vi "linearize_project.vi"() -> ()   [LabVIEW 2015]
uses:
  <vilib>/addons/Control Design/_Model Construction/Model Typedefs.llb/CD State Space Model (MIMO).ctl
  <vilib>/addons/Control Design/_Model Construction/Model Typedefs.llb/CD General Elements.ctl
  <vilib>/Simulation/Scripting/Companion Diagram/SimConfigNode/SimParams.ctl
  <vilib>/Simulation/Scripting/Companion Diagram/SimConfigNode/_simSolvers.ctl
  <vilib>/Simulation/Implementation/Shared/SIMSCR Execution Mode.ctl
  <vilib>/Simulation/Param Hierarchy/Typedefs/SIMPH Param Control Actions.ctl
  <vilib>/Simulation/Implementation/Shared/NILVSim_ParamChanged.vi
  <vilib>/Simulation/Implementation/Shared/NILVSIM_BeginStep.vi
  <vilib>/Simulation/DataSources/Implementation/NILVSim Step.llb/SIM Step (scalar).vi
  <vilib>/Simulation/ContinuousLinear/Implementation/NILVSim Transfer Function.llb/SIM Transfer Function Distributor (SISO CD).vi
  <vilib>/Simulation/ContinuousLinear/Implementation/NILVSim Transfer Function.llb/SIM Transfer Function Collector (SISO).vi
  <vilib>/Simulation/SignalDisplay/Implementation/NILVSim Time Waveform.llb/SIM Time Waveform (scalar).vi
  <vilib>/Simulation/Nonlinear/Implementation/NILVSim Saturation.llb/SIM Saturation (scalar).vi
  <vilib>/Simulation/Implementation/Shared/NILVSim_Manager.vi
  <vilib>/Utility/error.llb/Clear Errors.vi
  <vilib>/Simulation/Implementation/Shared/NILVSim_FinalizeModel.vi
  <vilib>/Simulation/Model Trim and Linearize/SIM Query Subsystem.llb/SIM Query Subsystem (Path).vi
  <vilib>/Simulation/Model Trim and Linearize/SIM Linearize.llb/SIM Linearize (Path).vi
  <vilib>/addons/Control Design/_Model Construction/Model Information.llb/Model Information SubVIs/cd_Get Matrices From SS Model.vi
  <vilib>/addons/Control Design/_Model Construction/Model Creation.llb/Model Creation SubVI/cd_Create State Space Model.vi
  <vilib>/addons/Control Design/_Model Conversions/Model Type.llb/Model Conversion SubVI/cd_Convert State-Space to Transfer Function Model.vi
  <vilib>/addons/Control Design/_Utility/Model Viewer.llb/Model Viewer SubVI/cd_Draw Transfer Function Equation (TF).vi
  <vilib>/addons/Control Design/_Model Construction/Model Creation.llb/Model Creation SubVI/cd_Create Transfer Function Model.vi
  <vilib>/addons/Control Design/_Model Interconnection/Model Interconnection.llb/Model Interconnection SubVI/cd_Add Models (TF and TF).vi
  <vilib>/Simulation/Implementation/Shared/SIM Unbundle Sim Info.vi
  <vilib>/Simulation/Implementation/Shared/NILVSim_Initialize.vi
  <vilib>/Simulation/Utility/Implementation/NILVSim Get Time and IsAcceptedStep.vi
  <vilib>/addons/control/pid/pid.llb/PID.vi
  <vilib>/addons/control/pid/pid.llb/PID (DBL).vi
  <vilib>/Simulation/Implementation/Shared/SIMSH Read Queue.vi
  <vilib>/Simulation/Implementation/Shared/NILVSim_GetModelError.vi
  <vilib>/Simulation/Implementation/Shared/SIM Bundle Sim Info.vi
  <vilib>/Simulation/Scripting/Companion Diagram/SimConfigNode/SimDog.xnode
  <vilib>/Simulation/Implementation/XNodeFramework/SimXNode/SimX.xnode
  <vilib>/addons/Control Design/_Model Construction/NI_LinSys_Model Information.lvlib
  <vilib>/addons/Control Design/_Model Construction/NI_LinSys_Model Creation.lvlib
  <vilib>/addons/Control Design/_Model Conversions/NI_CD_Model Type.lvlib
  <vilib>/addons/Control Design/_Utility/NI_CD_Model Viewer.lvlib
  <vilib>/addons/Control Design/_Model Interconnection/NI_CD_Model Interconnection.lvlib
  <vilib>/addons/Control Design/_Model Construction/NI_LinSys_Model Typedefs.lvlib
  <vilib>/addons/Control Design/_Model Construction/Model Typedefs.llb/CD Transfer Function Model (SISO).ctl
  <vilib>/addons/Control Design/_Model Construction/Model Typedefs.llb/CD Transfer Function Model (MIMO).ctl
  <vilib>/Simulation/ContinuousLinear/Implementation/NILVSim Transfer Function.llb/SIM Transfer Function (SISO CD).vi
  <vilib>/addons/control/pid/NI_PID_pid.lvlib
  <vilib>/Simulation/Implementation/Shared/NI_SIM_Implementation.lvlib
panel:
  in  "PID gains 2":T1={"proportional gain (Kc)"=1.0, "integral time (Ti, min)"=0.01, "derivative time (Td, min)"=0.0} {"derivative time (Td, min)" format="%.3f"; "integral time (Ti, min)" format="%.3f"; "proportional gain (Kc)" format="%.3f"}
  in  "set point 2":dbl
  in  "PID gains":T1={"proportional gain (Kc)"=1.0, "integral time (Ti, min)"=0.01, "derivative time (Td, min)"=0.0} {"derivative time (Td, min)" format="%.3f"; "integral time (Ti, min)" format="%.3f"; "proportional gain (Kc)" format="%.3f"}
  in  "set point1":dbl
  out "h2 2":waveform(dbl)(graph)
  out "h1 2":waveform(dbl)(graph)
  out "h2":waveform(dbl)(graph)
  out "h1":waveform(dbl)(graph)
  out "Equation":picture
  out "State-Space Model":T2 {"Transport Delay" format="%.2f"; "D" format="%#.2g"; "C" format="%#.2g"; "B" format="%#.6g"; "A" format="%#.6g"; "properties"."Sampling Time" format="%#.6p"; "properties"."Output Delays" format="%.4f"; "properties"."Input Delays" format="%.4f"}
  in  "Path":path
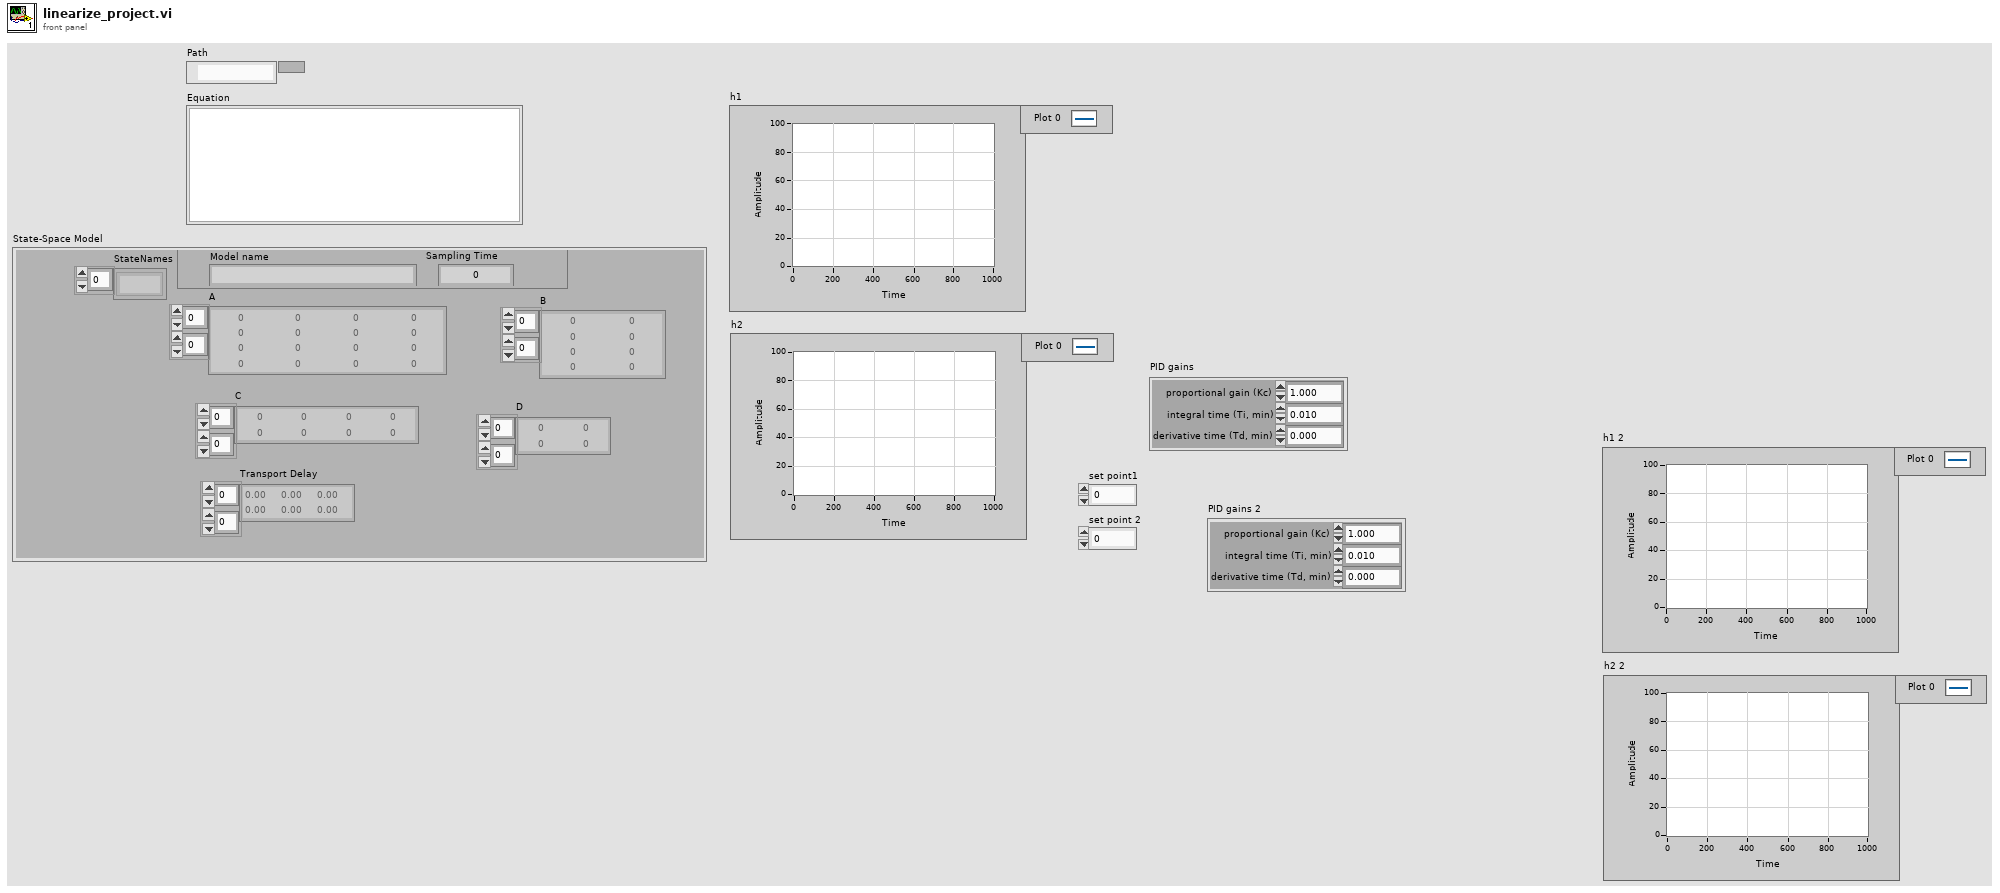
[diagram p1: front panel]
types:
  T1 = cluster{"proportional gain (Kc)":dbl, "integral time (Ti, min)":dbl, "derivative time (Td, min)":dbl}
  T2 = typedef "NI_LinSys_Model Typedefs.lvlib/CD State Space Model (MIMO).ctl" = cluster{"properties":T3, "A":dbl[][], "B":dbl[][], "C":dbl[][], "D":dbl[][], "StateNames":string[], "Transport Delay":dbl[][]}
  T3 = typedef "NI_LinSys_Model Typedefs.lvlib/CD General Elements.ctl" = cluster{"Model name":string, "Input names":string[], "Output names":string[], "Input Delays":dbl[], "Output Delays":dbl[], "Sampling Time":dbl, "Notes":string}
  T4 = typedef "SIM Trim or Lin Param.ctl" = cluster{"Name":string, "Value":dbl[], "Static Input?":bool, "Vector?":bool, "Fixed Size?":bool, "Fixed Value?":bool}
  T5 = typedef "NI_LinSys_Model Typedefs.lvlib/CD Transfer Function Model (MIMO).ctl" = cluster{"properties":T3, "transfer function(s)":T6[][]}
  T6 = typedef "NI_LinSys_Model Typedefs.lvlib/CD Transfer Function Model (SISO).ctl" = cluster{"Numerator":dbl[], "Denominator":dbl[], "delay":dbl}
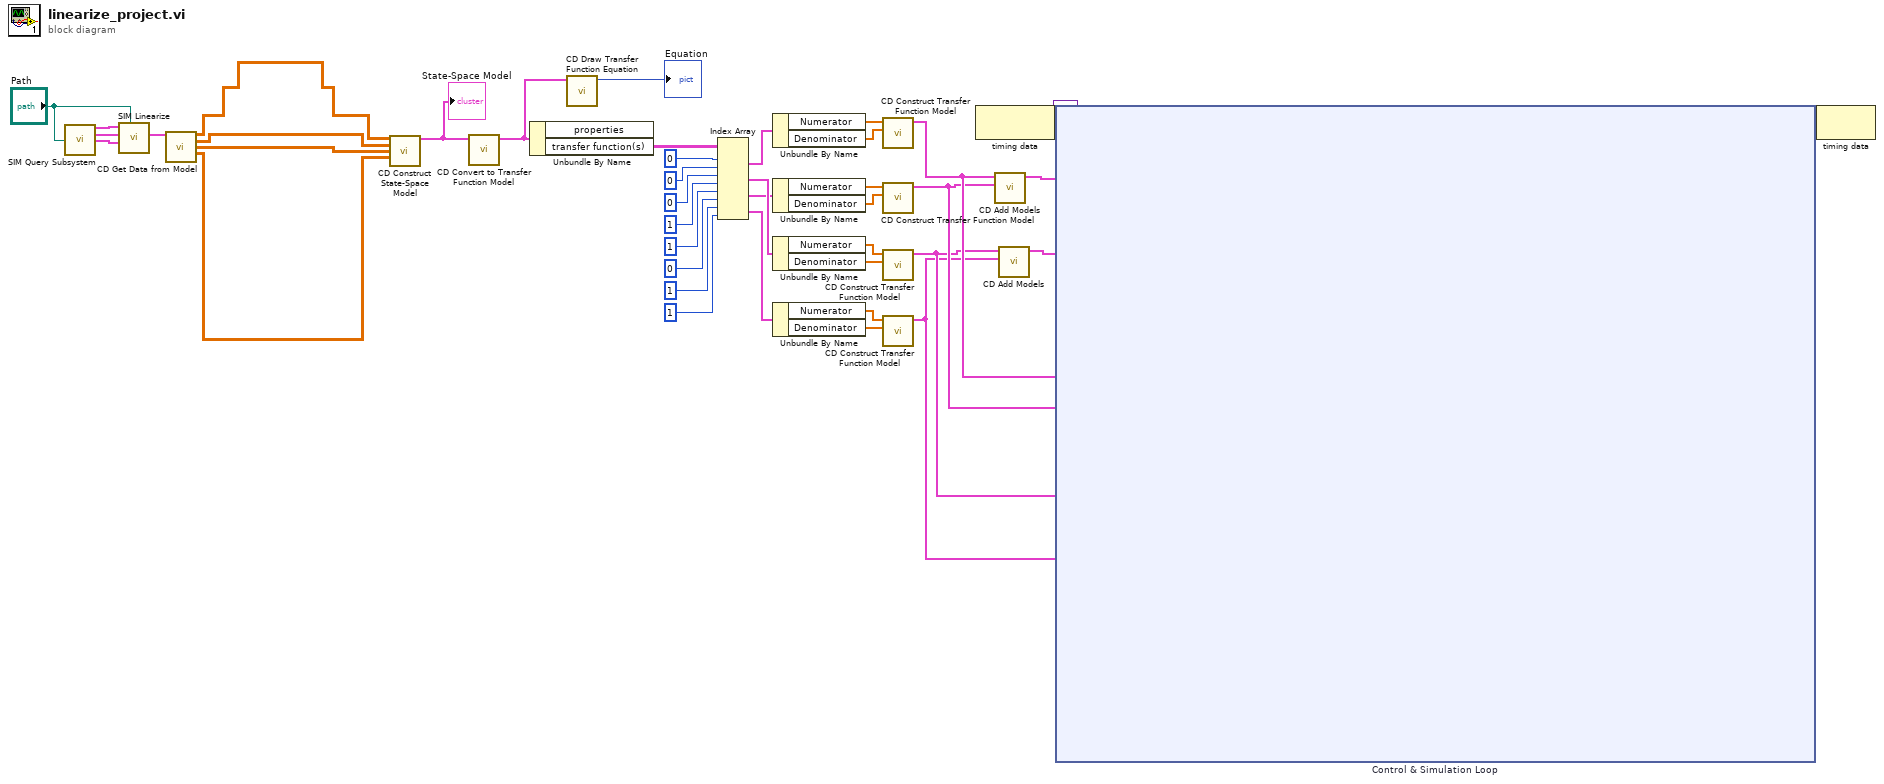
[diagram p0: block diagram]
diagram:
  n1 = call-poly <vilib>:"SIM Query Subsystem.vi"("Path"="Path") -> ("States"=w41:T4[], "Inputs"=w40:T4[], "Outputs"=w39:T4[])  [unwired: 10 in, 2 out]
  n2 = call-poly <vilib>:"SIM Linearize.vi"("Path"="Path", "Outputs"=w39, "Inputs"=w40, "States"=w41) -> ("State-Space Model"=w37:T2)  [unwired: 6 in, 1 out]
  n3 = call-poly <vilib>:"CD Get Data from Model.vi"("State-Space Model"=w37) -> ("Matrix A"=w6:dbl[][], "Matrix B"=w36:dbl[][], "Matrix C"=w5:dbl[][], "Matrix D"=w35:dbl[][])  [unwired: 10 in, 1 out]
  n4 = call-poly <vilib>:"CD Construct State-Space Model.vi"("A"=w6, "B"=w36, "C"=w5, "D"=w35) -> ("State-Space Model"=w34:T2)  [unwired: 10 in, 1 out]
  "State-Space Model" <- w34
  n5 = call-poly <vilib>:"CD Convert to Transfer Function Model.vi"("State-Space Model"=w34) -> ("Transfer Function Model"=w32:T5)  [unwired: 9 in, 1 out]
  n6 = Unbundle By Name(w32) -> ("transfer function(s)"=w31:T6[][])  [unwired: 1 out]
  n7 = call-poly <vilib>:"CD Draw Transfer Function Equation.vi"("Transfer Function Model"=w32) -> ("Equation"=→"Equation":picture)  [unwired: 8 in, 2 out]
  n8 = Index Array(array=w31, index (row) #1=0 ("index (row)"), index (col) #1=0 ("disabled index (col)"), index (row) #2=0 ("index (row)"), index (col) #2=1 ("disabled index (col)"), index (row) #3=1 ("index (row)"), index (col) #3=0 ("disabled index (col)"), index (row) #4=1 ("index (row)"), index (col) #4=1 ("disabled index (col)")) -> (element #1=w22:T6, element #2=w17:T6, element #3=w14:T6, element #4=w11:T6)
  n9 = Unbundle By Name(w22) -> ("Numerator"=w21:dbl[], "Denominator"=w20:dbl[])
  n10 = Unbundle By Name(w14) -> ("Numerator"=w16:dbl[], "Denominator"=w15:dbl[])
  n11 = Unbundle By Name(w17) -> ("Numerator"=w19:dbl[], "Denominator"=w18:dbl[])
  n12 = Unbundle By Name(w11) -> ("Numerator"=w13:dbl[], "Denominator"=w12:dbl[])
  n13 = call-poly <vilib>:"CD Construct Transfer Function Model.vi"("Denominator"=w20, "Numerator"=w21) -> ("Transfer Function Model"=w4:T5)  [unwired: 8 in, 1 out]
  n14 = call-poly <vilib>:"CD Construct Transfer Function Model.vi"("Denominator"=w15, "Numerator"=w16) -> ("Transfer Function Model"=w3:T5)  [unwired: 8 in, 1 out]
  n15 = call-poly <vilib>:"CD Construct Transfer Function Model.vi"("Denominator"=w18, "Numerator"=w19) -> ("Transfer Function Model"=w2:T5)  [unwired: 8 in, 1 out]
  n16 = call-poly <vilib>:"CD Construct Transfer Function Model.vi"("Denominator"=w12, "Numerator"=w13) -> ("Transfer Function Model"=w1:T5)  [unwired: 8 in, 1 out]
  n17 = node-c288() -> (w10:variant)  [unwired: 1 in]
  n18 = call-poly <vilib>:"CD Add Models.vi"("Model 2"=w3, "Model 1"=w4) -> ("Model Out"=w8:T5)  [unwired: 8 in, 1 out]
  n19 = call-poly <vilib>:"CD Add Models.vi"("Model 2"=w1, "Model 1"=w2) -> ("Model Out"=w7:T5)  [unwired: 8 in, 1 out]
  n20 = node-c254 "Control & Simulation Loop"(w10, w8, w7, w4, w3, w2, w1) -> (w9:variant)  [unwired: 1 out]
  n21 = node-c288(w9) -> ()  [unwired: 1 out]
